vi "Close.vi"(8 "error in":errorcluster, 11 "Red-y Read Write CFG in":refnum<class "Red-y Read Write CFG.lvclass">) -> (0 "error out":errorcluster, 3 "Red-y Read Write CFG out":refnum<class "Red-y Read Write CFG.lvclass">)   [LabVIEW 2023, in "Red-y Read Write CFG.lvclass"]
uses:
  Red-y Read Write CFG.lvclass
  Red-y Read Write CFG.lvclass/Red-y Read Write CFG.ctl
  CFG Target/CFG Target.lvclass
  Voegtlin_NI_SMART_Modbus_Drivers/Voegtlin_NI_SMART_Modbus_Drivers.lvlib
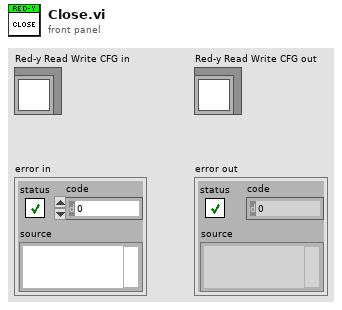
[diagram p1: front panel]
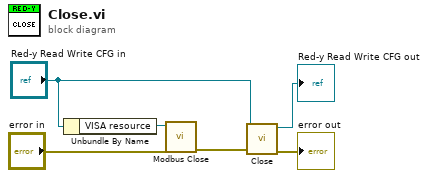
[diagram p0: block diagram]
diagram:
  n1 = Unbundle By Name("Red-y Read Write CFG in") -> ("VISA resource"=w2:refnum<visa-resource-name>)
  n2 = call "Modbus Close.vi"("error in (no error)"="error in", "VISA resource in"=w2) -> ("error out"=w1:errorcluster)  [unwired: 9 in]
  n3 = call-parent "Close.vi"("error in"=w1, "CFG Semaphore in"="Red-y Read Write CFG in") -> ("error out"=→"error out":errorcluster, "CFG Semaphore out"=→"Red-y Read Write CFG out":refnum<class "Red-y Read Write CFG.lvclass">)  [unwired: 8 in]
